vi "Prep for Plotting.vi"(9 "Quad Info":T1, 10 "Points":T2, 11 "Circle Info":cluster{"Radius":dbl, "Angle":dbl}) -> (1 "Length to Vertex":dbl, 2 "L2":dbl, 3 "XY Graph":cluster{"Array":cluster{dbl, dbl}[]}[](array[cluster]), 4 "Tangent Point":cluster{dbl, dbl})   [LabVIEW 2019]
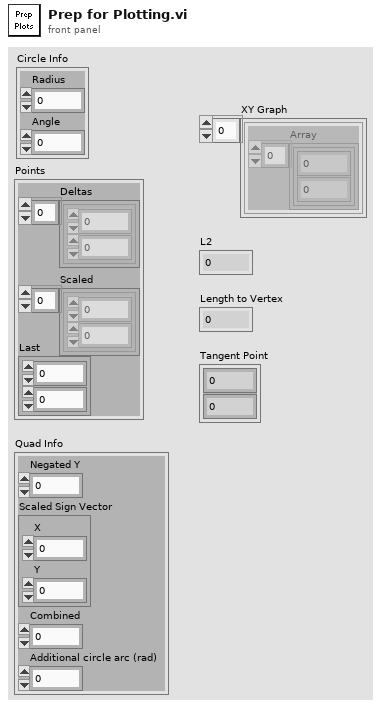
[diagram p1: front panel]
types:
  T1 = cluster{"Negated Y":i32, "Scaled Sign Vector":cluster{"X":dbl, "Y":dbl}, "Combined":i32, "Additional circle arc (rad)":dbl}
  T2 = cluster{"Deltas":cluster{dbl, dbl}[], "Scaled":cluster{dbl, dbl}[], "Last":cluster{dbl, dbl}}
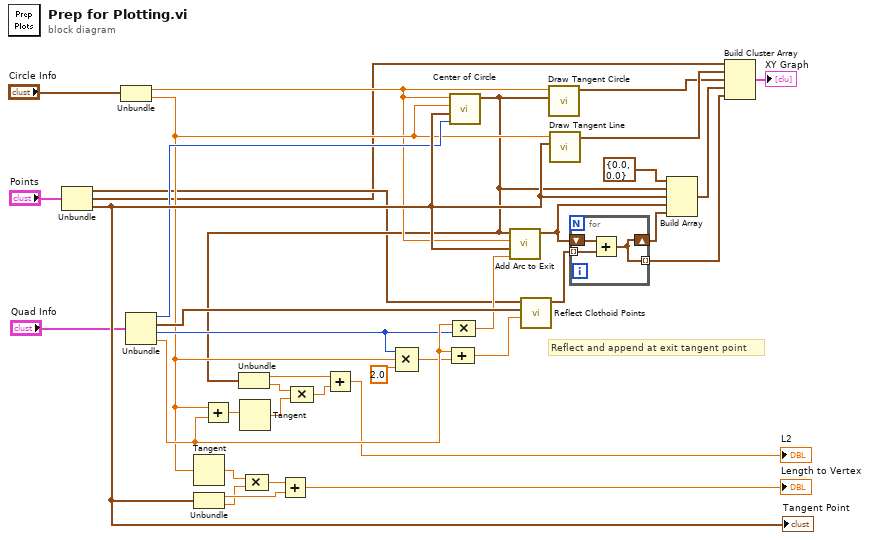
[diagram p0: block diagram]
diagram:
  # "Reflect and append at exit tangent point"
  n1 = Unbundle("Points") -> ("Deltas"=w2:cluster{dbl, dbl}[], "Scaled"=w1:cluster{dbl, dbl}[], "Last"=w37:cluster{dbl, dbl})
  "Tangent Point" <- w37
  n2 = Unbundle("Circle Info") -> ("Radius"=w27:dbl, "Angle"=w31:dbl)
  n3 = Unbundle("Quad Info") -> ("Negated Y"=w34:i32, "Scaled Sign Vector"=w33:cluster{"X":dbl, "Y":dbl}, "Combined"=w32:i32, "Additional circle arc (rad)"=w35:dbl)
  n4 = Tangent(1:w31) -> (0:w12:dbl)
  n5 = Unbundle(w37) -> (w15:dbl, w13:dbl)
  n6 = Add(x=w31, y=w35) -> (x+y=w20:dbl)
  n7 = Tangent(1:w20) -> (0:w21:dbl)
  n8 = Compound Arithmetic op=MULTIPLY(w12, w13) -> (w14:dbl)
  n9 = Add(x=w14, y=w15) -> (x+y=→"Length to Vertex":dbl)
  n10 = Compound Arithmetic op=MULTIPLY(w32, w31, 2.0) -> (w11:dbl)
  n11 = call "Center of Circle.vi"("Sign"=w34, "Tangent Point"=w37, "Tangent Angle"=w31, "Radius"=w27) -> ("Center Point"=w19:cluster{dbl, dbl})  [unwired: 7 in]
  n12 = Unbundle(w19) -> (w23:dbl, w22:dbl)
  n13 = Compound Arithmetic op=MULTIPLY(w22, w21) -> (w24:dbl)
  n14 = Add(x=w23, y=w24) -> (x+y=→"L2":dbl)
  n15 = Compound Arithmetic op=ADD(w35, w11) -> (w29:dbl)
  n16 = Compound Arithmetic op=MULTIPLY(w35, w32) -> (w30:dbl)
  n17 = call "Add Arc to Exit.vi"("Additional circle arc (rad)"=w30, "Tangent Point"=w37, "Radius"=w27, "Center Point"=w19) -> ("Blend Exit Point"=w8:cluster{dbl, dbl})  [unwired: 5 in, 2 out]
  n18 = call "Reflect Clothoid Points.vi"("Rotation"=w29, "Sign"=w33, "Points in"=w2) -> ("Points out"=w10:cluster{dbl, dbl}[])  [unwired: 8 in]
  n19 = call "Draw Tangent Circle.vi"("Cluster"=w19, "Numeric"=w27) -> ("Array"=w4:cluster{dbl, dbl}[])  [unwired: 9 in]
  n20 = call "Draw Tangent Line.vi"("Cluster"=w37, "Numeric"=w31) -> ("Array"=w7:cluster{dbl, dbl}[])  [unwired: 9 in]
  n21 = for {
    shift-right: [w38] -> w17
    shift-left: w8 -> [w39]
    tunnel: w10 -> [w40] mode=indexing
    tunnel: [w38] -> w5 mode=indexing
    n22 = Add(x=w39, y=w40) -> (x+y=w38:cluster{dbl, dbl})
  }
  n23 = Build Array(cluster{dbl, dbl} {0.0, 0.0}, w19, w37, w8, w17) -> (w6:cluster{dbl, dbl}[])
  n24 = Build Cluster Array(w1, w7, w4, w6, w5) -> (→"XY Graph":cluster{"Array":cluster{dbl, dbl}[]}[])
